vi "GetMessageParseError.vi"(8 "error in (no error)":errorcluster, 11 "body":variant) -> (0 "error out":errorcluster, 1 "error info":string, 2 "error code":i32)   [LabVIEW 2017]
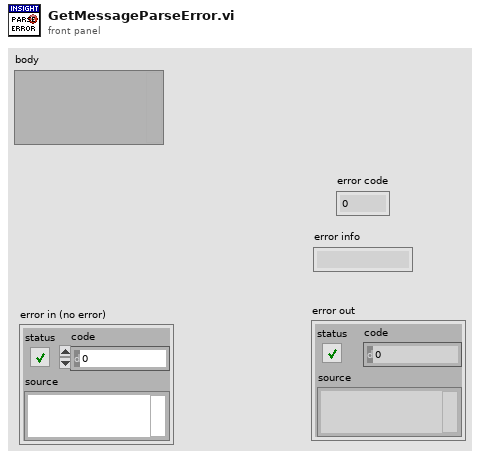
[diagram p1: front panel]
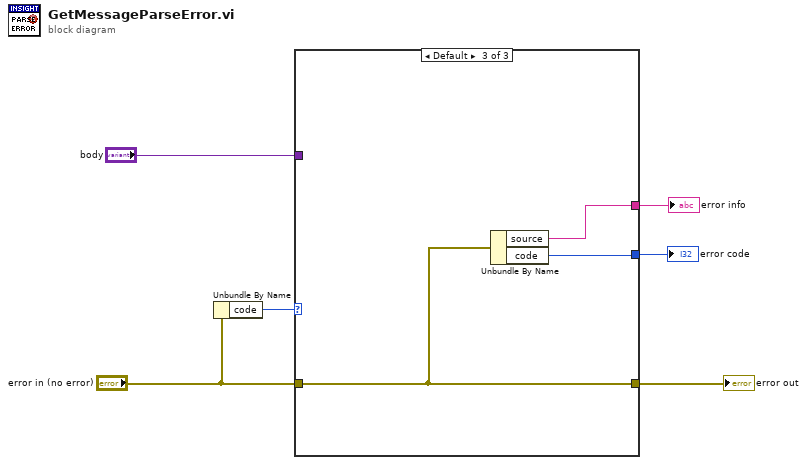
[diagram p0: block diagram]
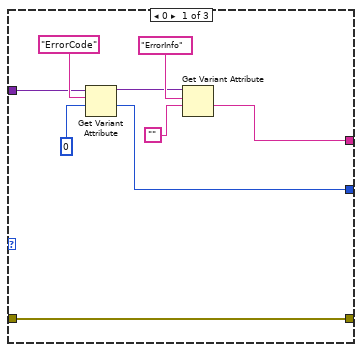
[diagram p2: hidden frame]
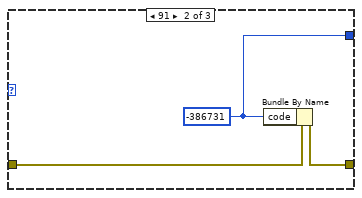
[diagram p3: hidden frame]
diagram:
  n1 = Unbundle By Name("error in (no error)") -> ("code"=w5:i32)
  n2 = case shown="Default" w5 {
    tunnel: "body" -> [w9 _ _]
    tunnel: [w7 w16 w20] -> w4
    tunnel: [w8 _ w19] -> w3
    tunnel: [w15 w17 w21] -> w2
    tunnel: "error in (no error)" -> [w15 w18 w21]
    frame 0 {
      n3 = Get Variant Attribute(Variant=w9, name="ErrorCode" ("Key"), default value (empty Variant)=0) -> (duplicate Variant=w12:variant, value=w7:i32)  [unwired: 1 in, 2 out]
      n4 = Get Variant Attribute(Variant=w12, name="ErrorInfo" ("Key"), default value (empty Variant)="") -> (value=w8:string)  [unwired: 1 in, 3 out]
    }
    frame 91 {
      w16 = -386731 ("code")
      n5 = Bundle By Name(cluster=w18, "code"=w16) -> (w17:errorcluster)
    }
    frame Default {
      n6 = Unbundle By Name(w21) -> ("source"=w19:string, "code"=w20:i32)
    }
  }
  "error code" <- w4
  "error info" <- w3
  "error out" <- w2
